vi "http server.vi"(9 "handler properties":T1={"max url size"=8000, "max header"=8000, "timeout ms"=5000, "max data size"=104857600}, 10 "connection handler pool size":i32=10, 11 "port":u16=80) -> (0 "error out":errorcluster)   [LabVIEW 2013]
uses:
  http server properties.ctl
  websocket/user plugin/websocket user plugin.lvclass
  HTTP responder/http responder.lvclass
  websocket/websocket upgrade handler.lvclass
panel:
  out "count":i32
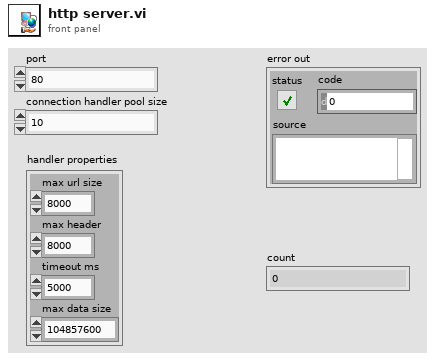
[diagram p1: front panel]
types:
  T1 = typedef "http server properties.ctl" = cluster{"max url size":i32, "max header":i32, "timeout ms":i32, "max data size":i32}
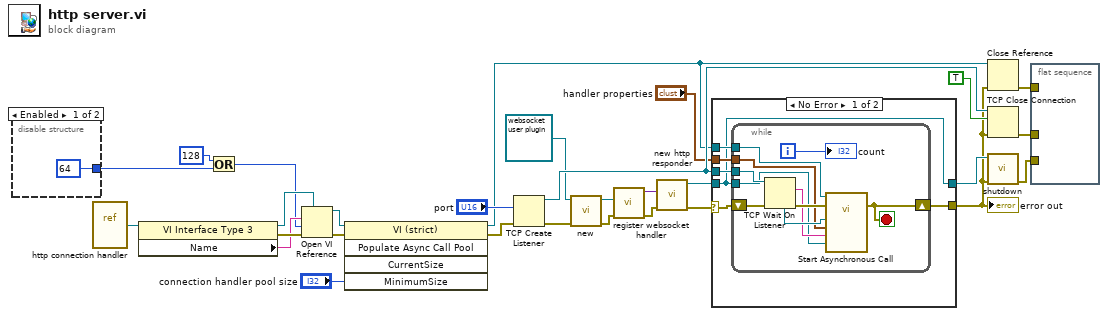
[diagram p0: block diagram]
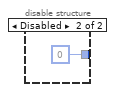
[diagram p2: hidden frame]
diagram:
  n1 = disable-structure shown="Enabled" {
    disable-tunnel: [64 ("options") 0 ("options")] -> w12
    frame Enabled {
    }
    frame Disabled {
    }
  }
  n2 = vi-ref "http connection handler.vi"() -> (w26:refnum<vi>)
  n3 = property class="VI Interface Type 3"(reference=w26) -> (reference out=w21:refnum<vi>, error out=w25:errorcluster, "Name"=w22:string)  [unwired: 1 in]
  n4 = Or(x=128 ("options"), y=w12) -> (x .or. y?=w20:i32)
  n5 = Open VI Reference(type specifier VI Refnum (for type only)=w21, vi path=w22, options=w20, error in (no error)=w25) -> (vi reference=w18:refnum<vi>, error out=w23:errorcluster)  [unwired: 2 in]
  n6 = invoke class="VI (strict)" method="Populate Async Call Pool"(reference=w18, error in=w23, "MinimumSize"="connection handler pool size") -> (reference out=w17:refnum<vi>, error out=w14:errorcluster)  [unwired: 2 in, 3 out]
  n7 = TCP Create Listener(8:w14, 10:"port") -> (0:w2:errorcluster, 3:w27:refnum<k5>)  [unwired: 3 in, 1 out]
  n8 = call-dynamic "new.vi"("error in"=w2, "websocket user plugin in"=refnum<class "websocket user plugin.lvclass"> refnum ("websocket user plugin")) -> ("error out"=w1:errorcluster, "websocket user plugin out"=w3:refnum<class "websocket user plugin.lvclass">)  [unwired: 8 in]
  n9 = call "register websocket handler.vi"("error in"=w1, "websocket user plugin"=w3) -> ("error out"=w5:errorcluster, "upgrade plugins out"=w6:variant)  [unwired: 8 in]
  n10 = call "new http responder.vi"("error in"=w5, "upgrade plugins"=w6) -> ("error out"=w11:errorcluster, "http responder out"=w10:refnum<class "http responder.lvclass">)  [unwired: 8 in]
  n11 = case shown="No Error" w11 {
    selector: w11 -> [w37 w49]
    tunnel: [w36 w49] -> w8
    tunnel: w27 -> [w35 _]
    tunnel: w17 -> [w34 _]
    tunnel: "handler properties" -> [w33 _]
    tunnel: w10 -> [w32 w48]
    tunnel: [w32 w48] -> w9
    frame No Error {
      n12 = while {
        shift-right: [w44] -> w36
        shift-left: w37 -> [w47]
        tunnel: w35 -> [w46]
        tunnel: w34 -> [w43]
        tunnel: w33 -> [w40]
        tunnel: w32 -> [w38]
        i -> [w39]
        stop <- w44 stop-if-true
        n13 = TCP Wait On Listener(8:w47, 11:w46) -> (0:w45:errorcluster, 2:w41:string, 4:w42:refnum<k5>)  [unwired: 2 in, 2 out]
        n14 = call-by-ref "Start Asynchronous Call"(reference=w43, error in=w45, "http responder"=w38, "remote address"=w41, "server properties"=w40, "connection"=w42) -> (error out=w44:errorcluster)  [unwired: 8 in, 1 out]
        "count" <- w39
      }
    }
    frame Error {
    }
  }
  "error out" <- w8
  n15 = Close Reference(reference=w17, error in (no error)=w8) -> (error out=w24:errorcluster)
  n16 = TCP Close Connection(connection ID=w27, abort (F)=TRUE, error in (no error)=w8) -> (error out=w28:errorcluster)  [unwired: 1 out]
  n17 = call "shutdown.vi"("error in"=w8, "http responder in"=w9) -> ("error out"=w7:errorcluster)  [unwired: 9 in]
  n18 = flat-sequence {
    tunnel: w28 -> [_]
    tunnel: w24 -> [_]
    tunnel: w7 -> [_]
    frame #0 {
    }
  }
